vi "Actor Core.vi"(8 "error in":errorcluster, 11 "Nested in":refnum<class "UI_Tree.lvclass">) -> (0 "error out":errorcluster, 3 "Actor out":refnum<class "Actor.lvclass">)   [LabVIEW 2021, in "UI_Tree.lvlib" / "UI_Tree.lvclass"]
doc: "(<B>Filename</B>: Actor Framework.lvlib:Actor.lvclass:Actor Core.vi)\n\nReceives messages to the actor, reacts to them, and initiates any error handling that may shut the actor down.\n\nDescendant classes may override this VI to append parallel tasks for the actor to complete while it handles messages. Overrides use the Call Parent Method node."
uses:
  UI_Tree.lvclass
  C:/Program Files (x86)/National Instruments/LabVIEW 2021/user.lib/John_Lib/AbstractActorTemplate/AbstractActorTemplate/UIActorTop.lvclass
  C:/Program Files (x86)/National Instruments/LabVIEW 2021/vi.lib/ActorFramework/Actor/Actor.lvclass
  <vilib>/ActorFramework/Actor/Actor.lvclass
  TopRef.ctl
  UI_Tree.lvclass/UI_Tree.ctl
  <vilib>/ActorFramework/Actor/Actor.lvclass/Actor.ctl
  <vilib>/ActorFramework/Message Enqueuer/Message Enqueuer.lvclass/Message Enqueuer.ctl
  <vilib>/ActorFramework/Message Enqueuer/Init from Existing Queue.vi
  <vilib>/ActorFramework/Message Enqueuer/Enqueue.vi
  <vilib>/ActorFramework/Stop Msg/Stop Msg.lvclass
  C:/Program Files (x86)/National Instruments/LabVIEW 2021/vi.lib/ActorFramework/Message/Message.lvclass
  <vilib>/ActorFramework/Message Priority Queue/Priority Enqueue.vi
  <vilib>/ActorFramework/Message Enqueuer/Message Enqueuer.lvclass
  <userlib>/John_Lib/AbstractActorTemplate/AbstractActorTemplate/UIActorTop.lvclass
panel:
  in  "Tree":string[](tree)
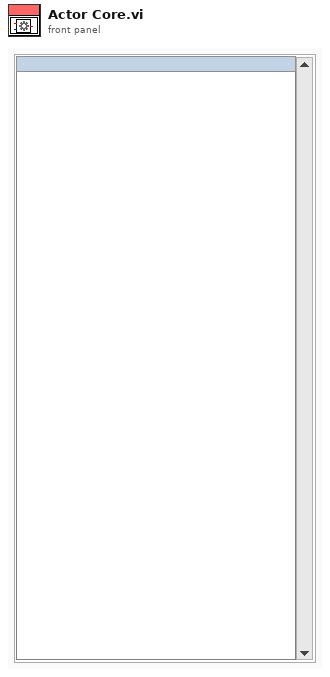
[diagram p1: front panel]
types:
  T1 = typedef "UI_Tree.lvlib/UI_Tree.lvclass/TopRef.ctl" = cluster{"Tree Refnum":refnum<vi>}
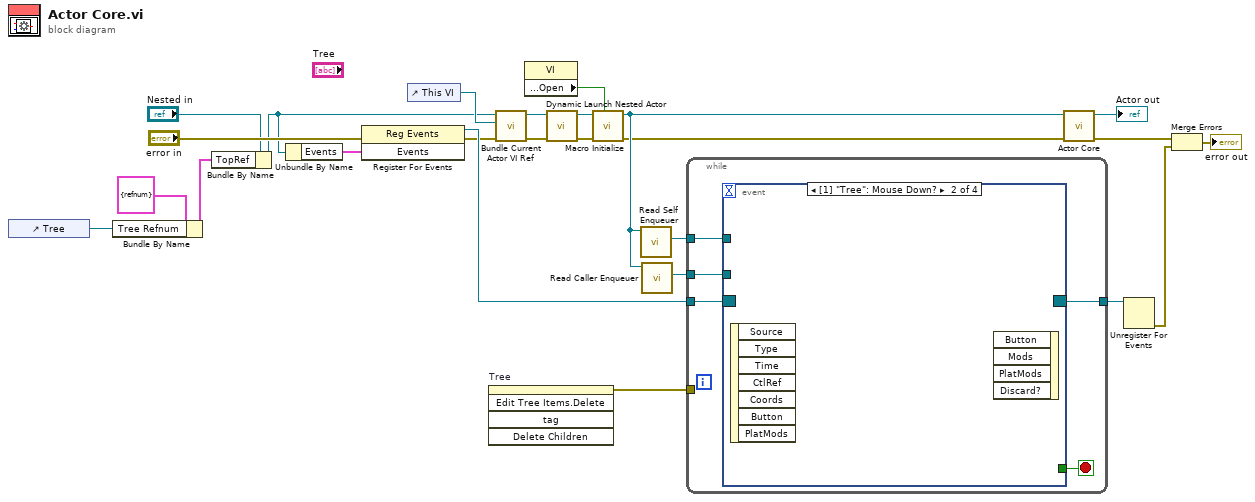
[diagram p0: block diagram]
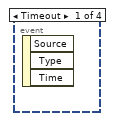
[diagram p2: hidden frame]
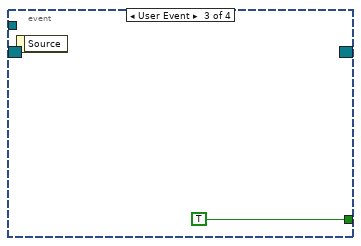
[diagram p3: hidden frame]
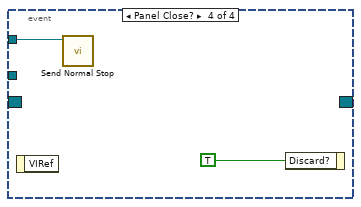
[diagram p4: hidden frame]
diagram:
  n1 = control-ref of="Tree"() -> (w1:refnum<vi>)
  n2 = Bundle By Name(cluster=T1 {"Tree Refnum"=refnum} ("TopRef"), "Tree Refnum"=w1) -> (w4:T1)
  n3 = Bundle By Name(cluster="Nested in", "TopRef"=w4) -> (w6:refnum<class "UI_Tree.lvclass">)
  n4 = Unbundle By Name(w6) -> ("Events"=w23:cluster{"Stop":refnum<user-event>})
  n5 = register-events ("Main Register for Events")(error in="error in", w23) -> (reference out=w24:refnum<event-registration>, error out=w9:errorcluster)  [unwired: 1 in]
  n6 = control-ref of="This VI"() -> (w7:refnum<vi>)
  n7 = invoke on="Tree" class="Tree (strict)" method="Edit Tree Items.Delete"() -> (error out=w3:errorcluster)  [unwired: 5 in, 4 out]
  n8 = call <userlib>:"Bundle Current Actor VI Ref.vi"("error in (no error)"=w9, "This VI"=w7, "UI ActorTop in"=w6) -> ("error out"=w8:errorcluster, "UI ActorTop in"=w10:refnum<class "UI_Tree.lvclass">)  [unwired: 5 in, 2 out]
  n9 = property class="VI"() -> ("Front Panel.Open"=w19:bool)  [unwired: 2 in, 2 out]
  n10 = call-dynamic "Dynamic Launch Nested Actor.vi"("error in (no error)"=w8, "UI ActorTop in"=w10) -> ("error out"=w20:errorcluster, "UI ActorTop out"=w21:refnum<class "UI_Tree.lvclass">)  [unwired: 8 in]
  n11 = call-dynamic "Macro Initialize.vi"("Front Panel Window:Open"=w19, "error in (no error)"=w20, "UI ActorTop in"=w21) -> ("error out"=w13:errorcluster, "UI ActorTop out"=w17:refnum<class "UI_Tree.lvclass">)  [unwired: 7 in]
  n12 = call <vilib>:"Read Self Enqueuer.vi"("Actor"=w17) -> ("Self Enqueuer"=w2:refnum<class "Message Enqueuer.lvclass">)  [unwired: 10 in]
  n13 = call <vilib>:"Read Caller Enqueuer.vi"("Actor"=w17) -> ("Caller Enqueuer"=w12:refnum<class "Message Enqueuer.lvclass">)  [unwired: 10 in]
  n14 = while {
    tunnel: w24 -> [w30]
    tunnel: [w28] -> w22
    tunnel: w2 -> [w27]
    tunnel: w12 -> [w26]
    tunnel: w3 -> [_]
    stop <- w29 stop-if-true
    n15 = event "UI Events" shown="[1] \"Tree\": Mouse Down?" {
      selector: w30 -> [_ _ _ _]
      dyn-events: [_ _ _ _] -> w28
      timeout: _ -> [_ _ _ _]
      tunnel: [_ _ TRUE _] -> w29
      tunnel: w27 -> [_ _ _ w32]
      tunnel: w26 -> [_ _ _ _]
      event Timeout {
        n16 = event-data() -> ()  [unwired: 1 in, 3 out]
      }
      event "Tree": Mouse Down? {
        n17 = event-data() -> ()  [unwired: 1 in, 7 out]
        n18 = event-data() -> ()  [unwired: 5 in, 1 out]
      }
      event User Event {
        n19 = event-data() -> ()  [unwired: 1 in, 1 out]
      }
      event Panel Close? {
        n20 = event-data() -> ()  [unwired: 1 in, 1 out]
        n21 = call <vilib>:"Send Normal Stop.vi"("Message Enqueuer"=w32) -> ()  [unwired: 10 in, 1 out]
        n22 = event-data("Discard?"=TRUE) -> ()  [unwired: 1 in, 1 out]
      }
    }
  }
  n23 = call-parent "Actor Core.vi"("error in"=w13, "Actor in"=w17) -> ("error out"=w15:errorcluster, "Actor out"=→"Actor out":refnum<class "Actor.lvclass">)  [unwired: 8 in]
  n24 = Unregister For Events(event registration refnum=w22) -> (error out=w16:errorcluster)  [unwired: 1 in]
  n25 = Merge Errors(w15, w16) -> (→"error out":errorcluster)
